vi "Store DVR history Mapping for circular history buffer.vi"(7 "Action":T1, 8 "error in":errorcluster, 9 "History DVR":refnum<data-value>, 10 "Device Name":string) -> (0 "error out":errorcluster, 1 "History DVR":refnum<data-value>, 2 "Found?":bool, 4 "All Names":string[](array[string]))   [LabVIEW 2015]
uses:
  typedefs/Data History.ctl
  typedefs/DVR Map Action.ctl
  <vilib>/Utility/error.llb/Error Cluster From Error Code.vi
  <vilib>/ErrorRing/Error Ring.xnode
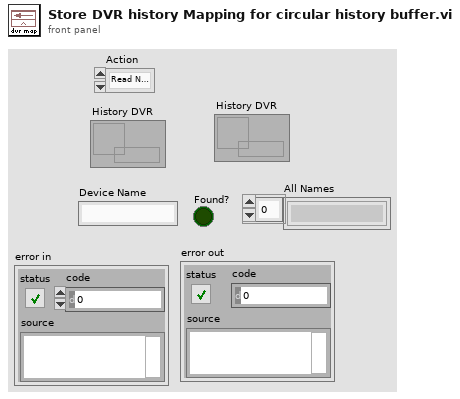
[diagram p1: front panel]
types:
  T1 = typedef "DVR Map Action.ctl" = enum16{"Read Names", "Write", "Read"}
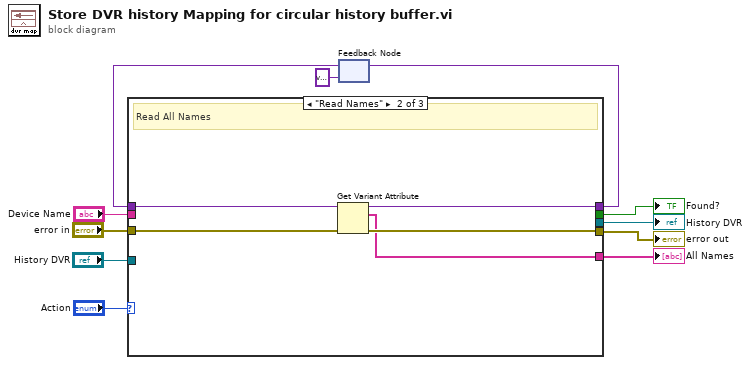
[diagram p0: block diagram]
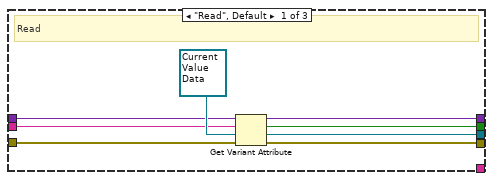
[diagram p2: hidden frame]
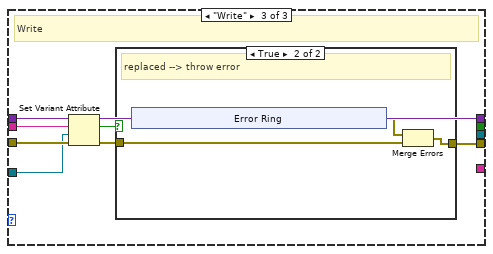
[diagram p3: hidden frame]
diagram:
  n1 = feedback #1(variant) -> (w6:variant)
  n2 = case shown="\"Read Names\"" "Action" {
    tunnel: "Device Name" -> [w18 _ w32]
    tunnel: [w17 _ _] -> w10
    tunnel: "error in" -> [w16 w24 w31]
    tunnel: [w15 w23 w25] -> w8
    tunnel: [w14 w22 w30] -> w7
    tunnel: w6 -> [w13 w21 w29]
    tunnel: [w12 _ _] -> w4
    tunnel: "History DVR" -> [_ _ w28]
    tunnel: [_ w20 _] -> w1
    frame "Read", Default {
      # "Read"
      n3 = Get Variant Attribute(Variant=w13, name=w18, default value (empty Variant)=refnum<data-value> refnum ("data value reference"), error in=w16) -> (duplicate Variant=w14:variant, found=w12:bool, value=w17:refnum<data-value>, error out=w15:errorcluster)
    }
    frame "Read Names" {
      # "Read All Names"
      n4 = Get Variant Attribute(Variant=w21, error in=w24) -> (duplicate Variant=w22:variant, names=w20:string[], error out=w23:errorcluster)  [unwired: 2 in, 1 out]
    }
    frame "Write" {
      # "Write"
      n5 = Set Variant Attribute(Variant=w29, name=w32, value=w28, error in=w31) -> (Variant out=w30:variant, replaced=w27:bool, error out=w26:errorcluster)
      n6 = case shown="True" w27 {
        tunnel: w26 -> [w33 w35]
        tunnel: [w33 w34] -> w25
        frame False {
        }
        frame True {
          # "replaced --> throw error"
          n7 = xnode "Error Ring"() -> ("error out"=w36:errorcluster)
          n8 = Merge Errors(w36, w35) -> (w34:errorcluster)
        }
      }
    }
  }
  "History DVR" <- w10
  "error out" <- w8
  "Found?" <- w4
  "All Names" <- w1
  n9 = feedback-in #1(w7) -> ()
